vi "writeToXML.vi"(8 "error in (no error)":errorcluster, 10 "ClassLabel":string, 11 "GuideTargetAbsorbOffset in":refnum<class "GuideTargetAbsorbOffset.lvclass">) -> (0 "error out":errorcluster, 2 "XML out":string, 3 "GuideTargetAbsorbOffset out":refnum<class "GuideTargetAbsorbOffset.lvclass">)   [LabVIEW 2022 SP3, in "TCSDataDefinitions.lvlib" / "TCSCommand.lvlib" / "OffsetCommands.lvlib" / "GuideTargetAbsorbOffset.lvclass"]
uses:
  GuideTargetAbsorbOffset.lvclass
  AbsorbOffset/AbsorbOffset.lvclass
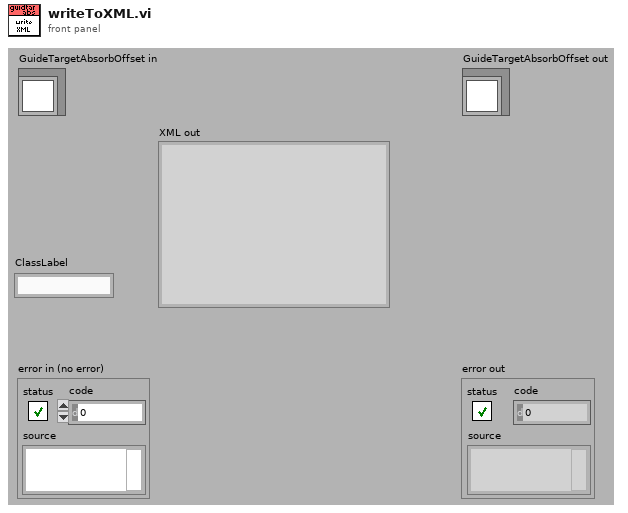
[diagram p1: front panel]
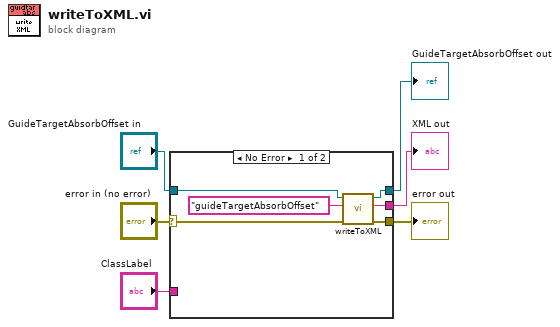
[diagram p0: block diagram]
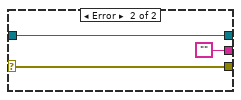
[diagram p2: hidden frame]
diagram:
  n1 = case shown="No Error" "error in (no error)" {
    selector: "error in (no error)" -> [w12 w15]
    tunnel: [w11 w15] -> w5
    tunnel: [w8 w14] -> w3
    tunnel: "GuideTargetAbsorbOffset in" -> [w9 w14]
    tunnel: [w10 ""] -> w2
    tunnel: "ClassLabel" -> [_ _]
    frame No Error {
      n2 = call-parent "writeToXML.vi"("error in (no error)"=w12, "ClassLabel"="guideTargetAbsorbOffset", "AbsorbOffset in"=w9) -> ("error out"=w11:errorcluster, "XML out"=w10:string, "AbsorbOffset out"=w8:refnum<class "GuideTargetAbsorbOffset.lvclass">)  [unwired: 6 in]
    }
    frame Error {
    }
  }
  "error out" <- w5
  "GuideTargetAbsorbOffset out" <- w3
  "XML out" <- w2
